vi "Transcriptor LabVIEW to C code 2.vi"(7 "vi path":path, 8 "Error In":errorcluster, 11 "Diagram in":refnum<vi>) -> (0 "Error Out":errorcluster, 1 "output cluster":T1, 2 "transcripted code":string, 3 "Diagram out":refnum<vi>)   [LabVIEW 2014]
panel:
  out "Cluster typedef[]":string[](array[string])
  out "FiringOrder":string[](array[string])
  out "Diagram wires declarations":string[](array[string])
  # "0. create definitions (ClusterConstant)\n1. get all wires and create their declarations\n2. if wires are connected to control or constant assign value to them\n3. translate elements of diagram by firing order\n4. assign values to outputs"
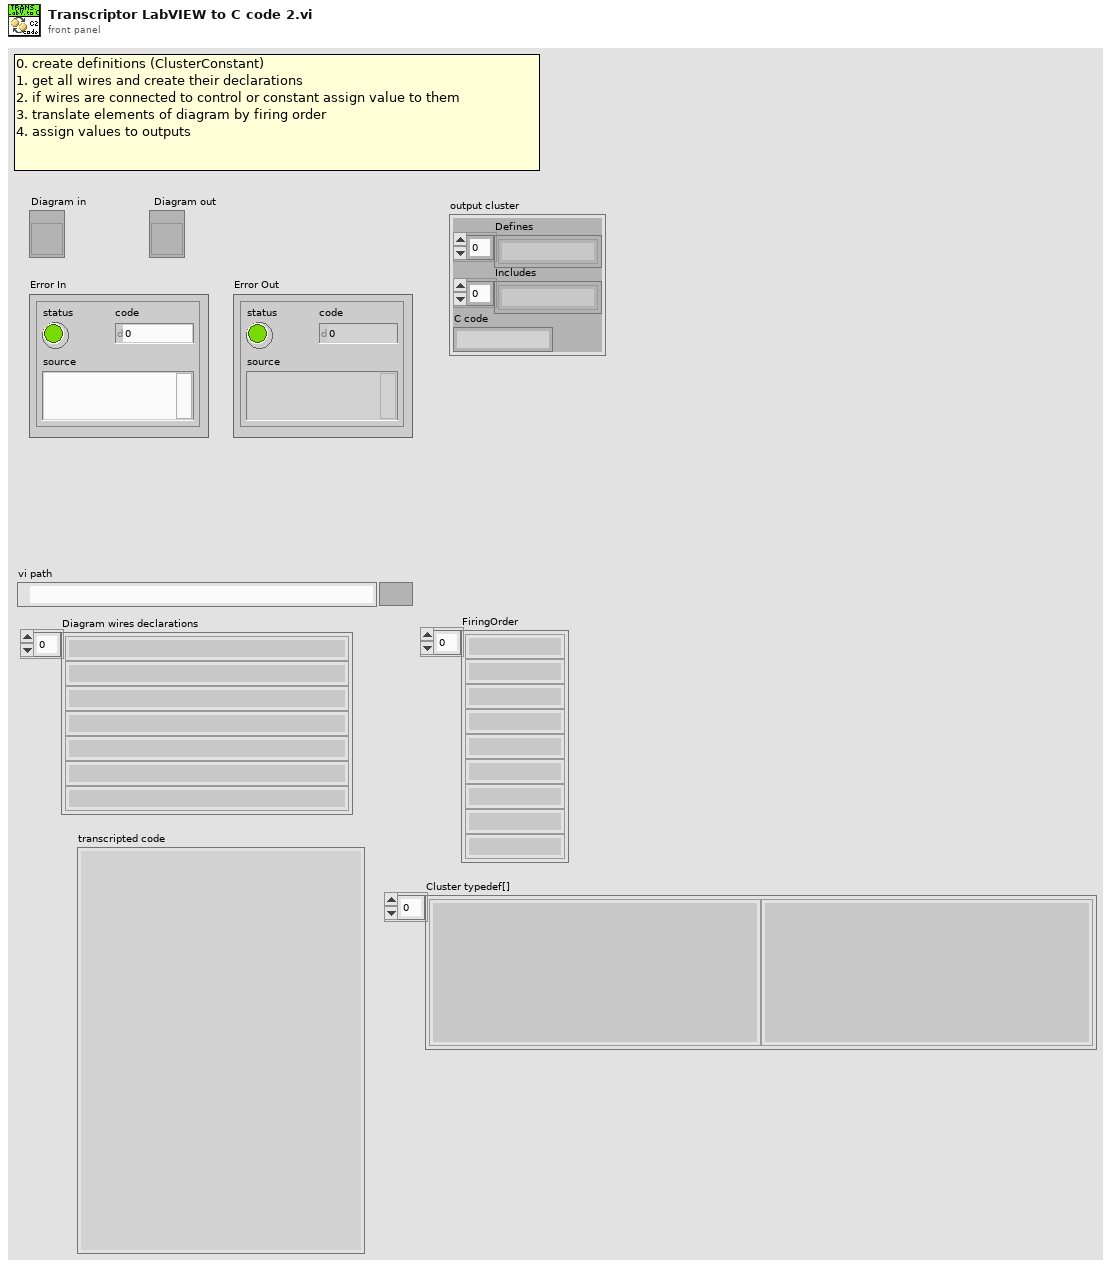
[diagram p1: front panel]
types:
  T1 = cluster{"Defines":string[], "Includes":string[], "C code":string}
  T2 = cluster{"wire labels":string[], "wire terminals datatypes":string[][]}
  T3 = cluster{"Defines":string[], "Includes":string[], "C code":string}[]
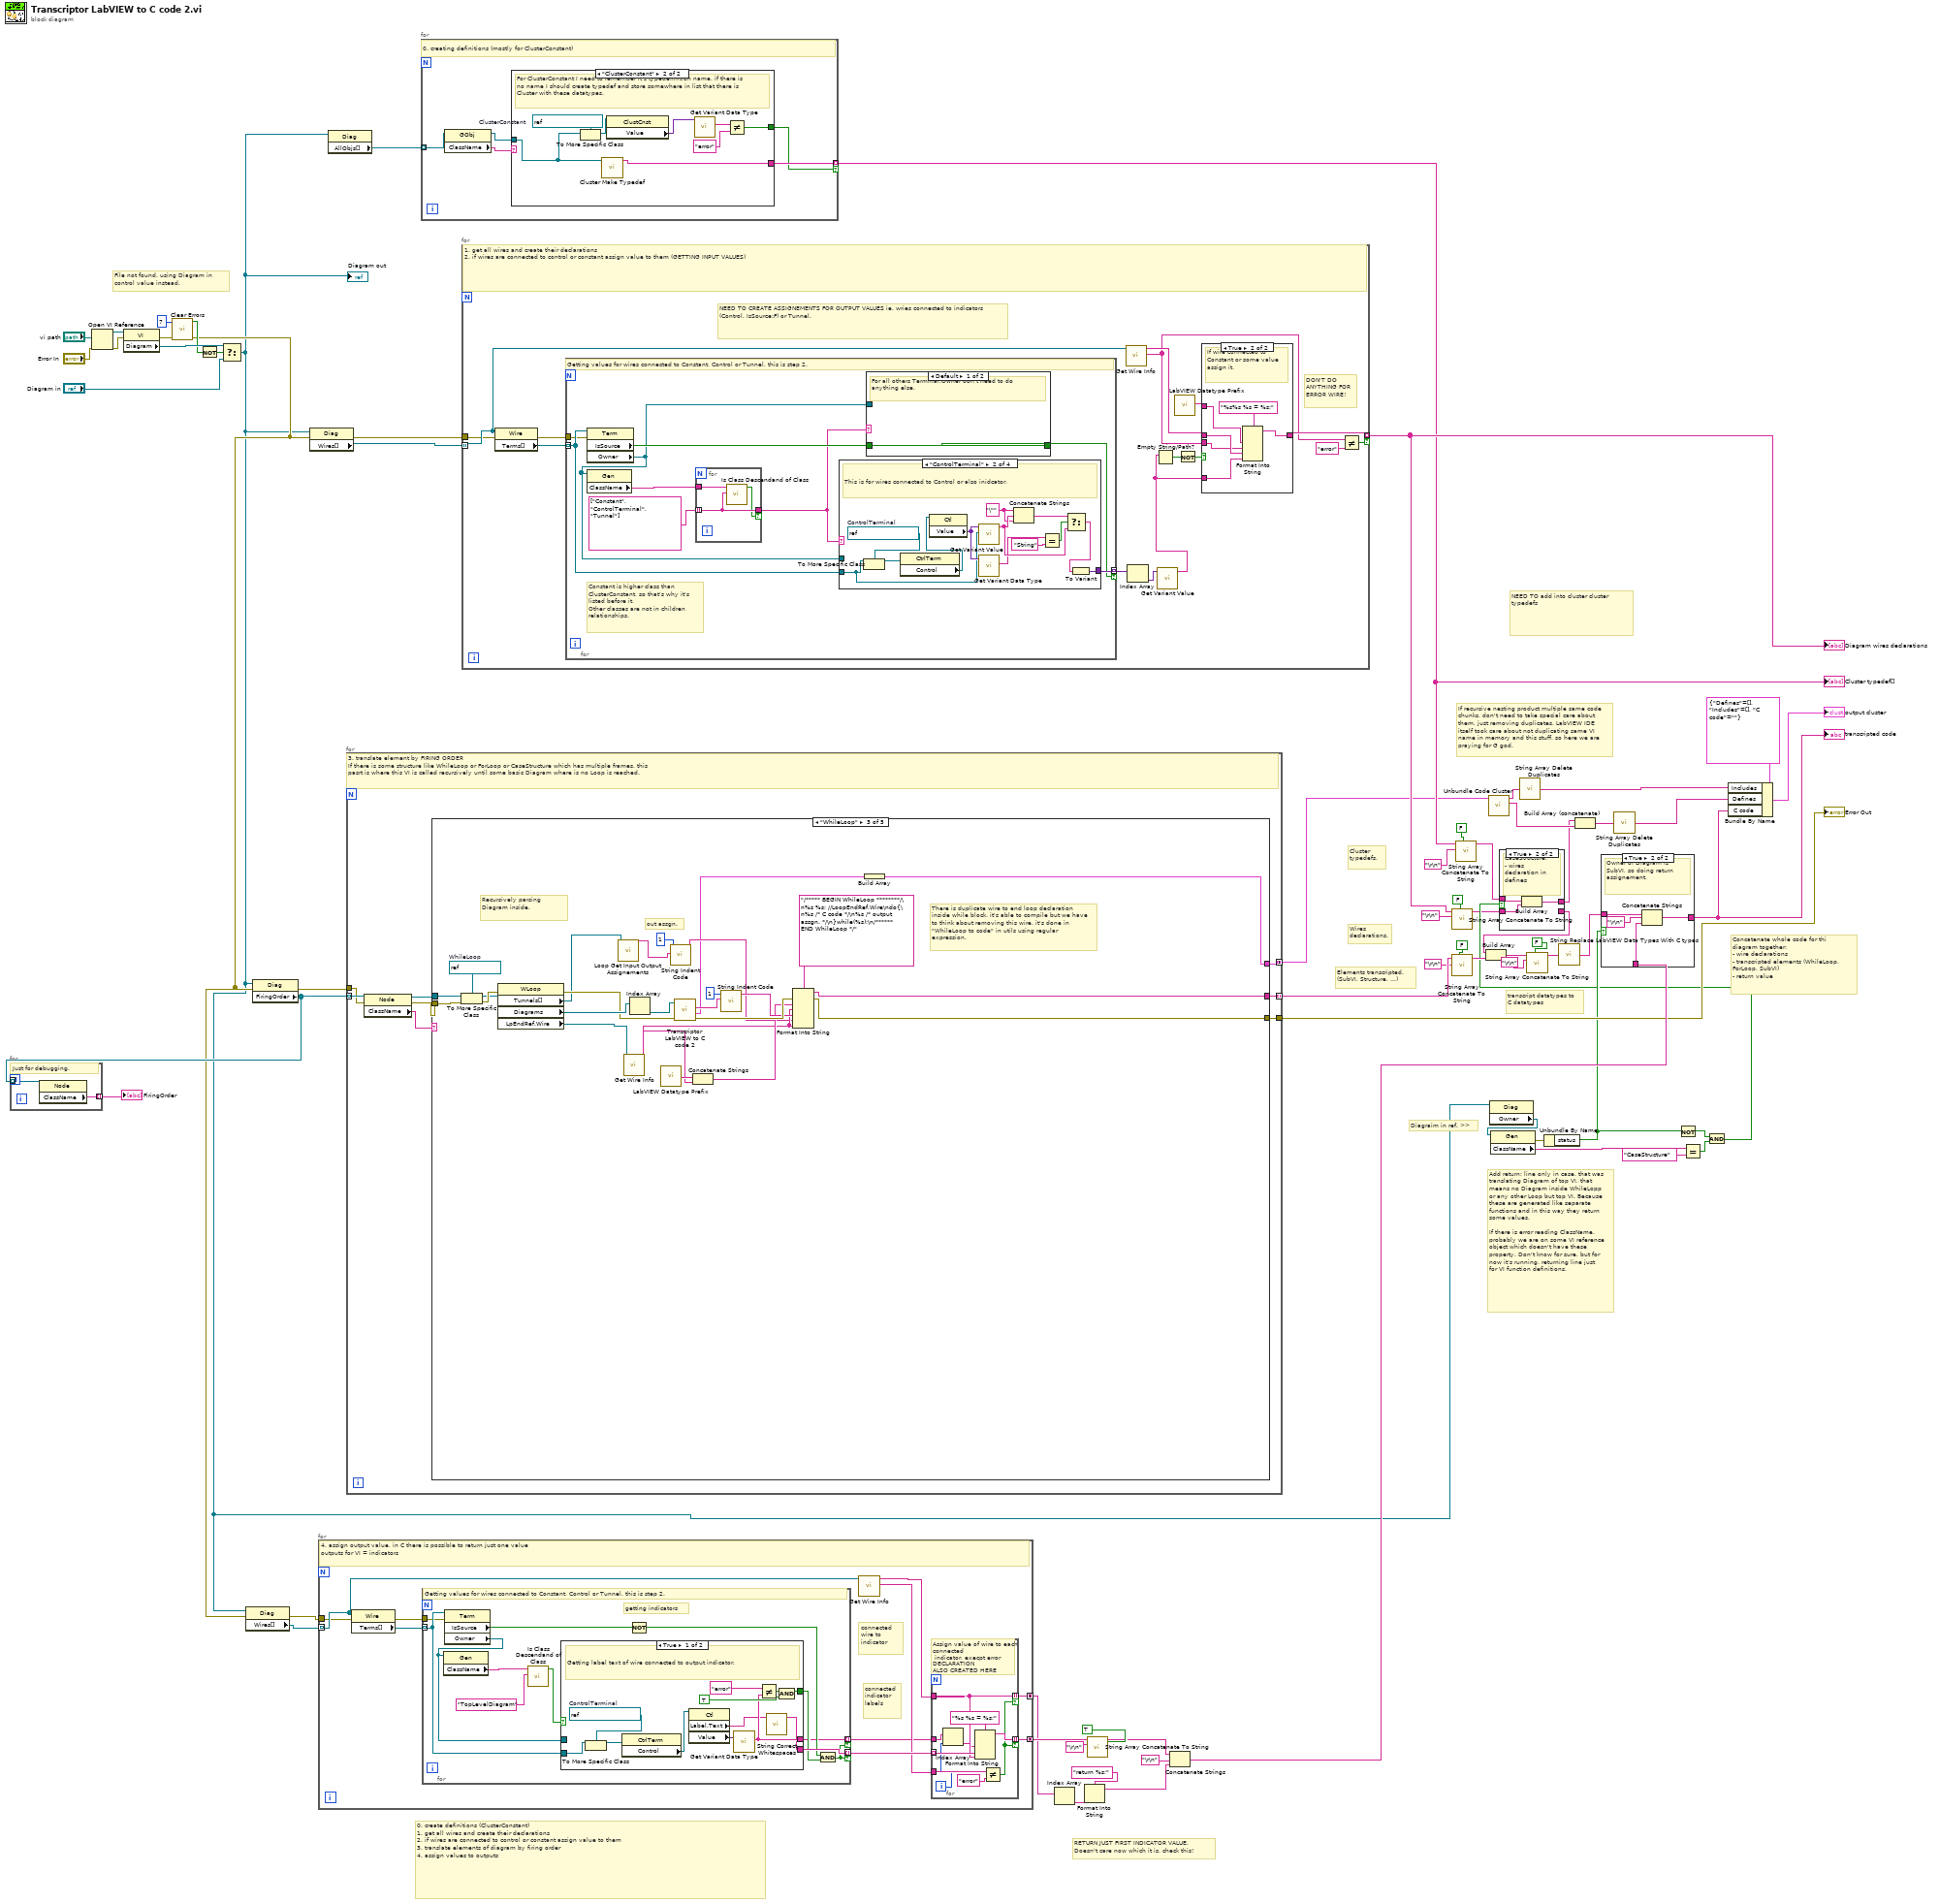
[diagram p0: block diagram]
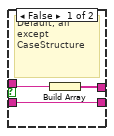
[diagram p2: hidden frame]
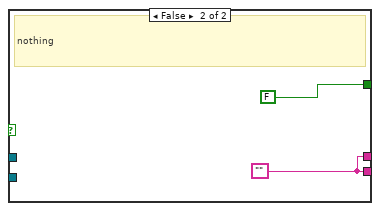
[diagram p4: hidden frame]
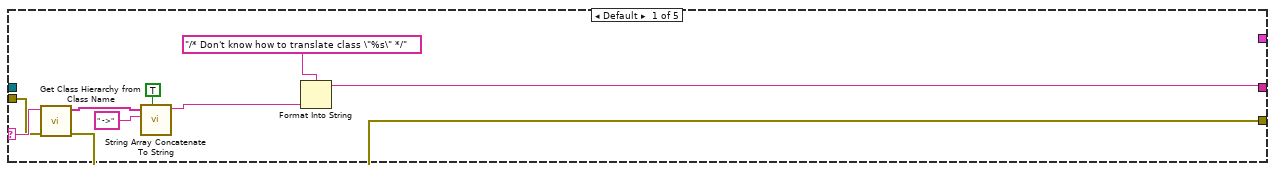
[diagram p6: hidden frame]
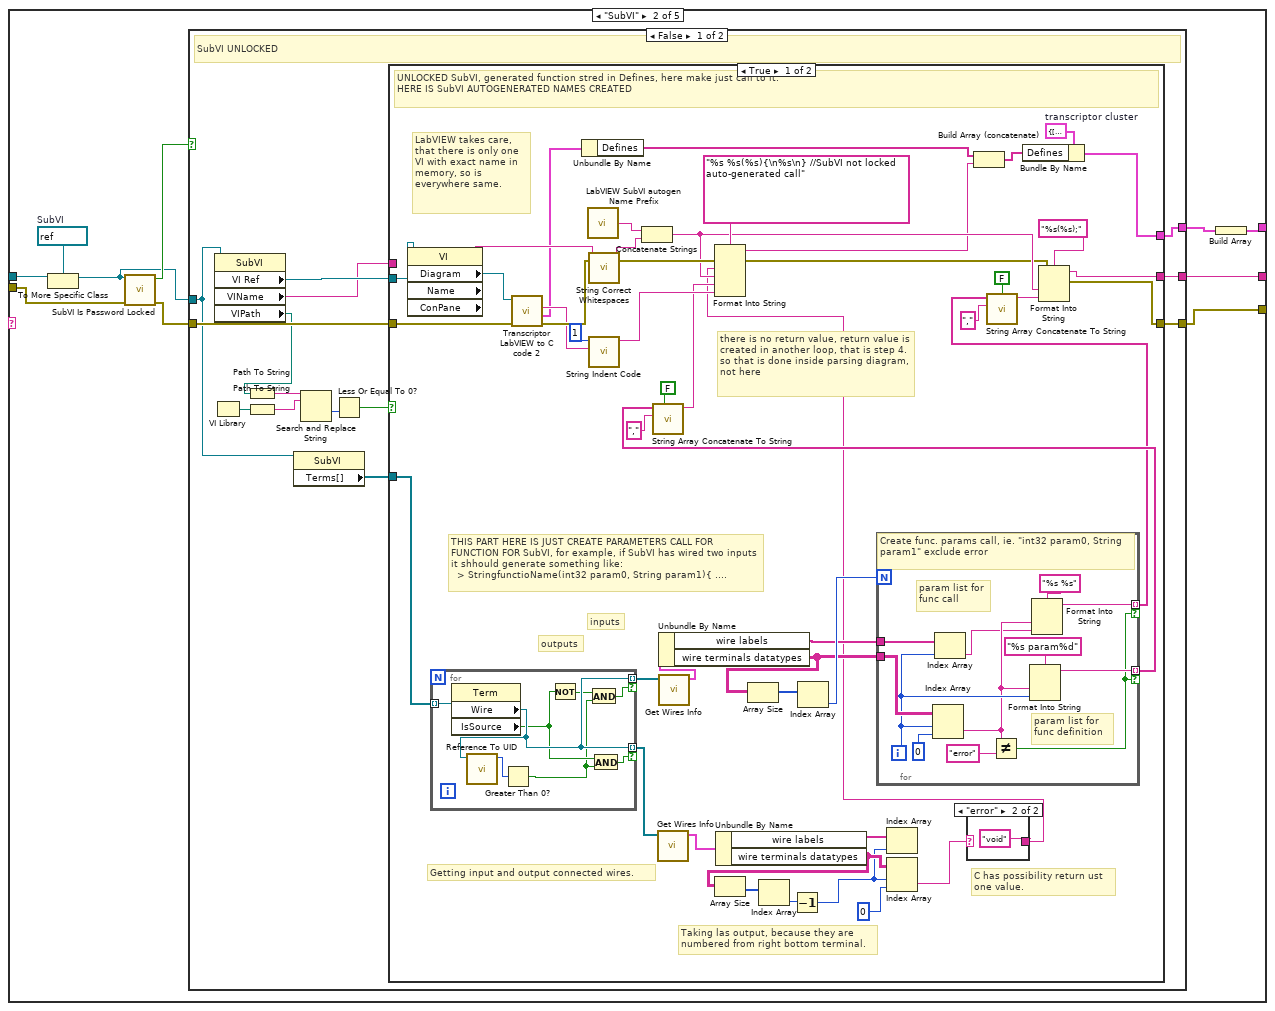
[diagram p7: hidden frame]
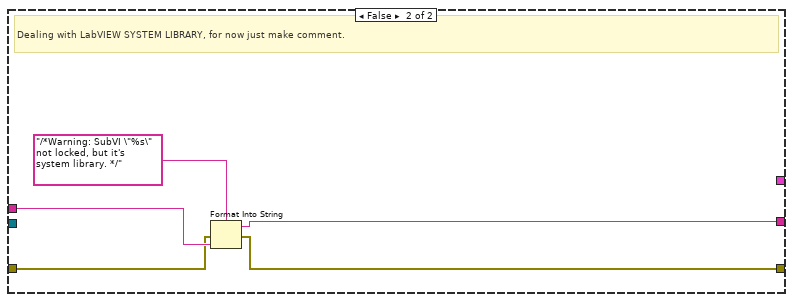
[diagram p9: hidden frame]
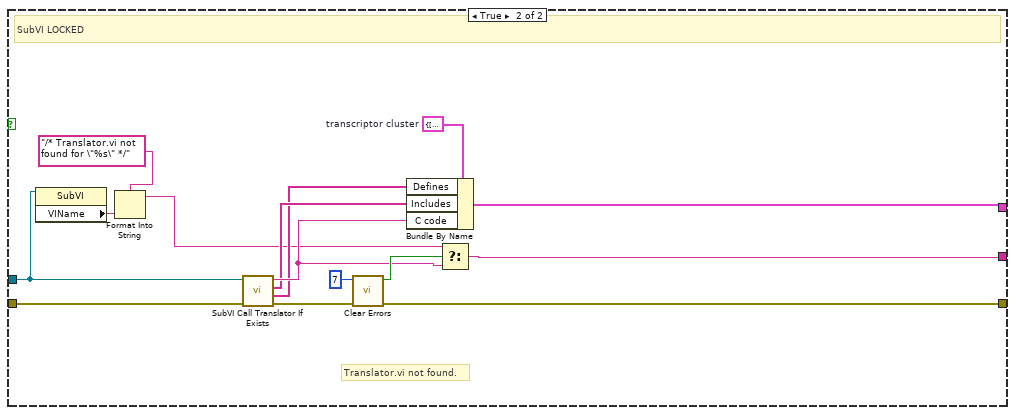
[diagram p10: hidden frame]
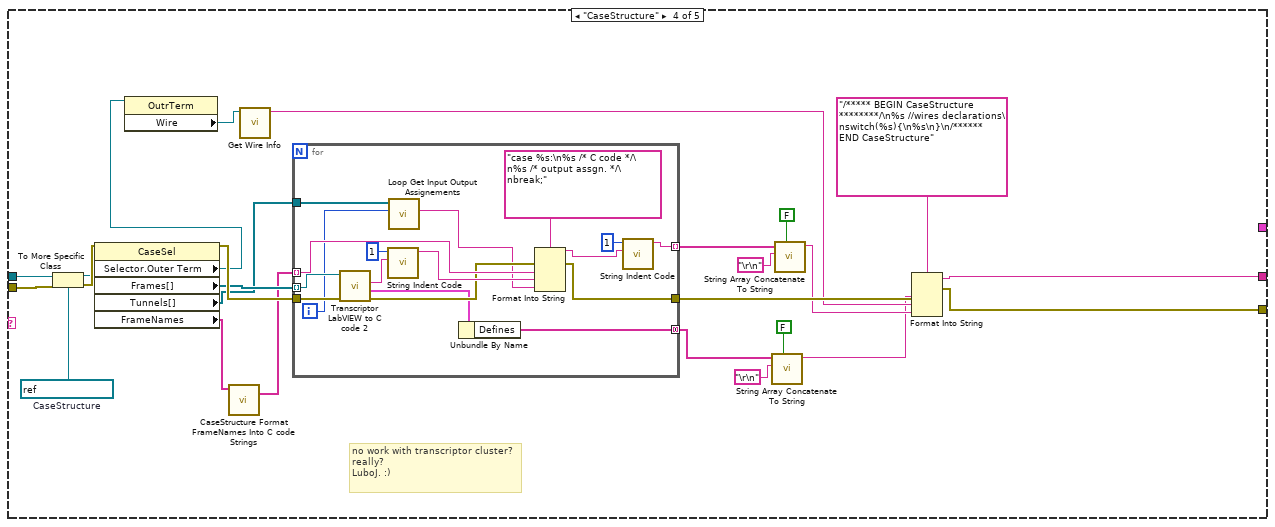
[diagram p11: hidden frame]
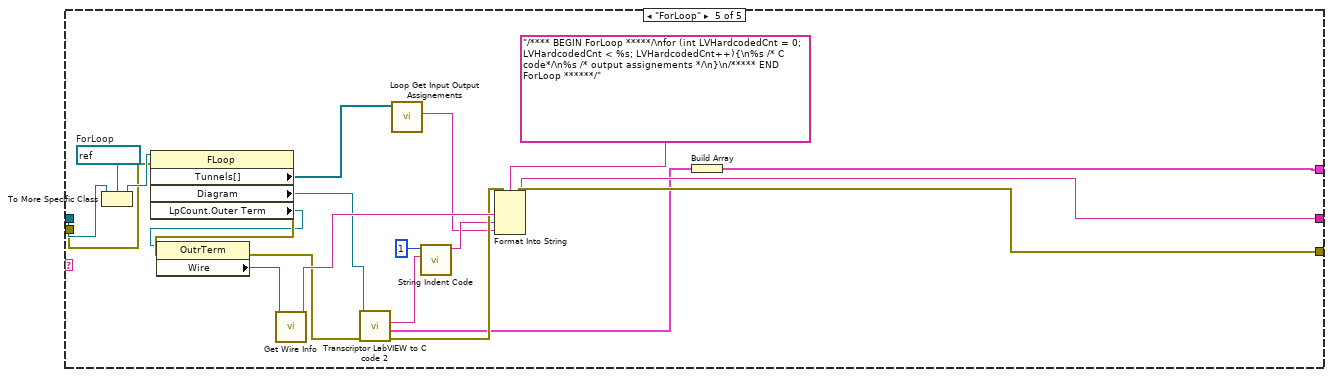
[diagram p12: hidden frame]
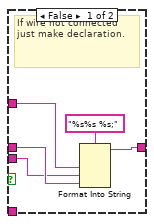
[diagram p13: hidden frame]
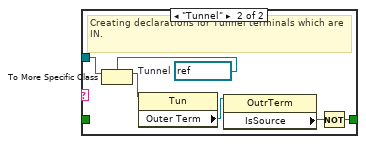
[diagram p14: hidden frame]
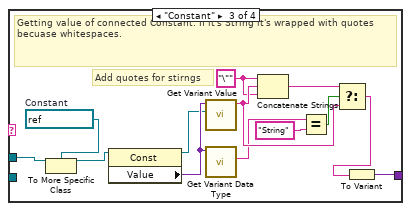
[diagram p16: hidden frame]
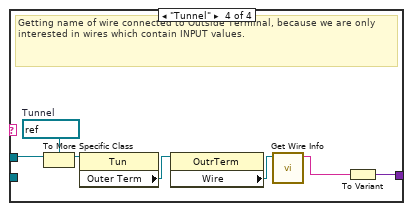
[diagram p17: hidden frame]
diagram:
  # "Diagraim in ref. >>"
  # "Add return; line only in case, that was translating Diagram of top VI, that means no Diagram inside WhileLopp or any other Loop but top VI. Because these are generated like separate functions and in this way they return some values.\n\nIf there is error reading ClassName, probably we are on some VI reference object which doesn't have these property. Don't know for sure, but for now it's running, returning line just for VI function definitions."
  # "RETURN JUST FIRST INDICATOR VALUE.\nDoesn't care now which it is, check this!"
  # "Concatenate whole code for thi diagram together:\n- wire declarations\n- transcripted elements (WhileLoop, ForLoop, SubVI)\n- return value"
  # "0. create definitions (ClusterConstant)\n1. get all wires and create their declarations\n2. if wires are connected to control or constant assign value to them\n3. translate elements of diagram by firing order\n4. assign values to outputs"
  # "If recursive nesting product multiple same code chunks, don't need to take special care about them, just removing duplicates, LabVIEW IDE itself took care about not duplicating same VI name in memory and this stuff, so here we are praying for G god."
  # "NEED TO add into cluster cluster typedefs"
  # "transcript datatypes to C datatypes"
  # "Elements transcripted.\n(SubVI, Structure, ...)"
  # "Wires declarations."
  # "Cluster typedefs."
  # "File not found, using Diagram in control value instead."
  n1 = Open VI Reference(vi path="vi path", error in (no error)="Error In") -> (vi reference=w66:refnum<vi>, error out=w65:errorcluster)  [unwired: 4 in]
  n2 = property class="VI"(reference=w66, error in=w65) -> (error out=w50:errorcluster, "Diagram"=w54:refnum<vi>)  [unwired: 1 out]
  n3 = call <vilib>:"Clear Errors.vi"("error in (no error)"=w50, "specific error code to clear (0: all)"=7) -> ("error out"=w29:errorcluster, "specific error cleared?"=w48:bool)  [unwired: 4 in]
  n4 = Not(x=w48) -> (.not. x?=w47:bool)
  n5 = Select(t=w54, s=w47, f="Diagram in") -> (s? t:f=w13:refnum<vi>)
  "Diagram out" <- w13
  n6 = property class="Diag"(reference=w13, error in=w29) -> (error out=w30:errorcluster, "Wires[]"=w31:refnum<vi>[])  [unwired: 1 out]
  n7 = property class="Diag"(reference=w13, error in=w29) -> (error out=w62:errorcluster, "FiringOrder"=w52:refnum<vi>[])  [unwired: 1 out]
  n8 = for {
    tunnel: w52 -> [w69] mode=indexing
    tunnel: [w68] -> w51 mode=indexing
    # "Just for debugging."
    n9 = property class="Node"(reference=w69) -> ("ClassName"=w68:string)  [unwired: 1 in, 2 out]
  }
  "FiringOrder" <- w51
  n10 = property class="Diag"(reference=w13, error in=w29) -> (error out=w63:errorcluster, "Wires[]"=w64:refnum<vi>[])  [unwired: 1 out]
  n11 = for {
    tunnel: w31 -> [w78] mode=indexing
    tunnel: w30 -> [w77]
    tunnel: [w73] -> w25 mode=concatenating
    tunnel: [w72] -> w23 mode=concatenating
    # "connected indicator labels"
    # "connected wire to indicator"
    # "4. assign output value, in C there is possible to return just one value\noutputs for VI = indicators"
    n12 = property class="Wire"(reference=w78, error in=w77) -> (error out=w76:errorcluster, "Terms[]"=w79:refnum<vi>[])  [unwired: 1 out]
    n13 = for {
      tunnel: w79 -> [w101] mode=indexing
      tunnel: [w94] -> w75 mode=indexing if=w90
      tunnel: w76 -> [w100]
      tunnel: [w91] -> w70 mode=indexing if=w90
      # "getting indicators"
      # "Getting values for wires connected to Constant, Control or Tunnel, this is step 2."
      n14 = property class="Term"(reference=w101, error in=w100) -> ("IsSource"=w99:bool, "Owner"=w98:refnum<vi>)  [unwired: 2 out]
      n15 = property class="Gen"(reference=w98) -> ("ClassName"=w97:string)  [unwired: 1 in, 2 out]
      n16 = call "Is Class Descendand of Class.vi"("Parent ClassName"="TopLevelDiagram", "ClassName"=w97) -> ("is Class descendant?"=w95:bool)  [unwired: 8 in, 1 out]
      n17 = case shown="True" w95 {
        tunnel: w98 -> [_ _]
        tunnel: w101 -> [w110 _]
        tunnel: [w102 w114] -> w94
        tunnel: [w105 FALSE] -> w92
        tunnel: [w104 w114] -> w91
        frame True {
          w113 = refnum<vi> refnum  # ControlTerminal
          # "Getting label text of wire connected to output indicator."
          n18 = To More Specific Class(target class=w113, reference=w110) -> (specific class reference=w112:refnum<vi>)  [unwired: 1 in, 1 out]
          n19 = property class="CtrlTerm"(reference=w112) -> ("Control"=w111:refnum<vi>)  [unwired: 1 in, 2 out]
          n20 = property class="Ctl"(reference=w111) -> ("Label.Text"=w103:string, "Value"=w109:variant)  [unwired: 1 in, 2 out]
          n21 = call "Get Variant Data Type.vi"("Variant in"=w109) -> ("first data type"=w104:string)  [unwired: 9 in, 1 out]
          n22 = Not Equal?(x="error", y=w104) -> (x != y?=w107:bool)
          n23 = call "String Correct Whitespaces.vi"("String in"=w103) -> ("String out"=w102:string)  [unwired: 10 in]
          n24 = And(x=w107, y=TRUE) -> (x .and. y?=w105:bool)
        }
        frame False {
          w114 = ""
          # "nothing"
        }
      }
      n25 = Not(x=w99) -> (.not. x?=w93:bool)
      n26 = And(x=w93, y=w92) -> (x .and. y?=w90:bool)
    }
    n27 = call "Get Wire Info.vi"("Wire"=w78) -> ("wire datatype"=w71:string, "wire label"=w74:string)  [unwired: 9 in]
    n28 = for {
      tunnel: w75 -> [w88] mode=indexing
      tunnel: w74 -> [w86]
      tunnel: [w87] -> w73 mode=indexing if=w83
      tunnel: [w86] -> w72 mode=indexing if=w83
      tunnel: w71 -> [w85]
      tunnel: w70 -> [w81]
      i -> [w82]
      # "Assign value of wire to each connected\n indicator, execpt error\nDECLARATION\nALSO CREATED HERE"
      n29 = Index Array(array=w81, index=w82) -> (element=w80:string)
      n30 = Format Into String(format string="%s %s = %s;", w80, w88, w86) -> (resulting string=w87:string)  [unwired: 2 in, 1 out]
      n31 = Not Equal?(x=w85, y="error" ("format string")) -> (x != y?=w83:bool)
    }
  }
  n32 = property class="Diag"(reference=w13) -> ("AllObjs[]"=w40:refnum<vi>[])  [unwired: 1 in, 2 out]
  n33 = for {
    tunnel: w52 -> [w123] mode=indexing
    tunnel: w62 -> [w121]
    tunnel: [w119] -> w61 mode=indexing
    tunnel: [w117] -> w14
    tunnel: [w116] -> w15 mode=concatenating
    # "3. translate element by FIRING ORDER\nIf there is some structure like WhileLoop or ForLoop or CaseStructure which has multiple frames, this\npasrt is where this VI is called recursively until some basic Diagram where is no Loop is reached."
    n34 = property class="Node"(reference=w123, error in=w121) -> (reference out=w120:refnum<vi>, error out=w118:errorcluster, "ClassName"=w122:string)
    n35 = case shown="\"WhileLoop\"" w122 {
      selector: w122 -> [w130 _ _ _ _]
      tunnel: w120 -> [_ w142 w271 w278 w334]
      tunnel: [w131 w138 w263 w291 w324] -> w119
      tunnel: w118 -> [w125 w137 w267 w294 w331]
      tunnel: [w124 w135 w261 w289 w325] -> w117
      tunnel: [_ w133 w254 _ w315] -> w116
      frame Default {
        n36 = call <vilib>:"Get Class Hierarchy from Class Name.vi"("error in (no error)"=w125, "Class Name"=w130) -> ("error out"=w124:errorcluster, "Class Hierarchy"=w128:string[])  [unwired: 8 in]
        n37 = call "String Array Concatenate To String.vi"("insert last delimiter?"=TRUE, "Delimiter char"=" ->", "Array String In"=w128) -> ("String"=w126:string)  [unwired: 8 in]
        n38 = Format Into String(format string="/* Don't know how to translate class \"%s\" */", w126) -> (resulting string=w131:string)  [unwired: 2 in, 1 out]
      }
      frame "SubVI" {
        w141 = refnum<vi> refnum  # SubVI
        n39 = To More Specific Class(target class=w141, reference=w142) -> (specific class reference=w139:refnum<vi>)  [unwired: 1 in, 1 out]
        n40 = call "SubVI Is Password Locked.vi"("Error In"=w137, "SubVI ref"=w139) -> ("Error Out"=w136:errorcluster, "isPasswordLocked?"=w140:bool)  [unwired: 8 in]
        n41 = case shown="False" w140 {
          tunnel: w139 -> [w145 w235]
          tunnel: [w154 w242] -> w138
          tunnel: w136 -> [w156 w241]
          tunnel: [w153 w240] -> w135
          tunnel: [w143 w231] -> w134
          frame False {
            # "SubVI UNLOCKED"
            n42 = VI Library() -> (path=w150:path)
            n43 = property class="SubVI"(reference=w145) -> ("VI Ref"=w155:refnum<vi>, "VIName"=w152:string, "VIPath"=w151:path)  [unwired: 1 in, 2 out]
            n44 = Path To String(path=w151) -> (string=w149:string)
            n45 = Path To String(path=w150) -> (string=w148:string)
            n46 = property class="SubVI"(reference=w145) -> ("Terms[]"=w144:refnum<vi>[])  [unwired: 1 in, 2 out]
            n47 = Search and Replace String(input string=w149, search string=w148) -> (number of replacements=w147:i32)  [unwired: 6 in, 3 out]
            n48 = Less Or Equal To 0?(x=w147) -> (x <= 0?=w146:bool)
            n49 = case shown="True" w146 {
              tunnel: w156 -> [w203 w226]
              tunnel: w155 -> [w186 _]
              tunnel: [w201 w229] -> w154
              tunnel: [w188 w228] -> w153
              tunnel: w152 -> [_ w227]
              tunnel: [w202 _] -> w143
              tunnel: w144 -> [w179 _]
              frame True {
                w159 = T1 {"Defines"=[], "Includes"=[], "C code"=""}  # transcriptor cluster
                # "THIS PART HERE IS JUST CREATE PARAMETERS CALL FOR FUNCTION FOR SubVI, for example, if SubVI has wired two inputs it shhould generate something like:\n  > StringfunctioName(int32 param0, String param1){ ...."
                # "there is no return value, return value is created in another loop, that is step 4.\nso that is done inside parsing diagram, not here"
                # "Taking las output, because they are numbered from right bottom terminal."
                # "outputs"
                # "inputs"
                # "Getting input and output connected wires."
                # "C has possibility return ust one value."
                # "LabVIEW takes care, that there is only one VI with exact name in memory, so is everywhere same."
                # "UNLOCKED SubVI, generated function stred in Defines, here make just call to it.\nHERE IS SubVI AUTOGENERATED NAMES CREATED"
                n50 = property class="VI" props=["Diagram", "Name", "ConPane"](reference=w186) -> ("Diagram"=w187:refnum<vi>, "Name"=w198:string)  [unwired: 1 in, 3 out]
                n51 = for {
                  tunnel: [w223] -> w177 mode=indexing if=w220
                  tunnel: [w223] -> w178 mode=indexing if=w221
                  tunnel: w179 -> [w225] mode=indexing
                  n52 = property class="Term"(reference=w225) -> ("Wire"=w223:refnum<vi>, "IsSource"=w219:bool)  [unwired: 1 in, 2 out]
                  n53 = call "Reference To UID.vi"("Reference"=w223) -> ("UID"=w224:i32)  [unwired: 10 in]
                  n54 = Greater Than 0?(x=w224) -> (x > 0?=w218:bool)
                  n55 = Not(x=w219) -> (.not. x?=w222:bool)
                  n56 = And(x=w222, y=w218) -> (x .and. y?=w221:bool)
                  n57 = And(x=w219, y=w218) -> (x .and. y?=w220:bool)
                }
                n58 = call "Transcriptor LabVIEW to C code 2.vi"("Error In"=w203, "Diagram in"=w187) -> ("Error Out"=w199:errorcluster, "output cluster"=w158:T1, "transcripted code"=w197:string)  [unwired: 6 in, 1 out]
                n59 = Unbundle By Name(w158) -> ("Defines"=w157:string[])
                n60 = call "LabVIEW SubVI autogen Name Prefix.vi"() -> ("datatype prefix"=w194:string)
                n61 = call "String Correct Whitespaces.vi"("String in"=w198) -> ("String out"=w193:string)  [unwired: 10 in]
                n62 = call "String Indent Code.vi"("complete code"=w197, "actual nested level"=1) -> ("indented code"=w183:string)  [unwired: 9 in]
                n63 = Concatenate Strings(w194, w193) -> (w192:string)
                n64 = call "Get Wires Info.vi"("connected\nwires refs."=w177) -> ("output cluster 2"=w181:T2)  [unwired: 10 in]
                n65 = call "Get Wires Info.vi"("connected\nwires refs."=w178) -> ("output cluster 2"=w176:T2)  [unwired: 10 in]
                n66 = Unbundle By Name(w176) -> ("wire labels"=w171:string[], "wire terminals datatypes"=w173:string[][])
                n67 = Unbundle By Name(w181) -> ("wire labels"=w180:string[], "wire terminals datatypes"=w163:string[][])
                n68 = Array Size(array=w163) -> (size(s)=w162:i32[])
                n69 = Array Size(array=w173) -> (size(s)=w175:i32[])
                n70 = Index Array(array=w162) -> (element=w161:i32)  [unwired: 1 in]
                n71 = Decrement(x=w161) -> (x-1=w160:i32)
                n72 = Index Array(array=w175) -> (element=w174:i32)  [unwired: 1 in]
                n73 = for {
                  N: w174 -> [_]
                  tunnel: w173 -> [w217]
                  tunnel: [w214] -> w172 mode=indexing if=w207
                  tunnel: w171 -> [w212]
                  tunnel: [w206] -> w167 mode=indexing if=w207
                  i -> [w211]
                  # "param list for\nfunc call"
                  # "param list for\nfunc definition"
                  # "Create func. params call, ie. \"int32 param0, String param1\" exclude error"
                  n74 = Index Array(array=w217, index (row)=w211, index (col)=0 ("disabled index (col)")) -> (element=w209:string)
                  n75 = Index Array(array=w212, index=w211) -> (element=w208:string)
                  n76 = Not Equal?(x=w209, y="error") -> (x != y?=w207:bool)
                  n77 = Format Into String(format string="%s param%d", w209, w211) -> (resulting string=w214:string)  [unwired: 2 in, 1 out]
                  n78 = Format Into String(format string="%s %s", w209, w208) -> (resulting string=w206:string)  [unwired: 2 in, 1 out]
                }
                n79 = call "String Array Concatenate To String.vi"("insert last delimiter?"=FALSE, "Delimiter char"=",", "Array String In"=w172) -> ("String"=w182:string)  [unwired: 8 in]
                n80 = Index Array(array=w180, index=w160) -> ()  [unwired: 1 out]
                n81 = Index Array(array=w163, index (row)=w160, index (col)=0 ("index (row)")) -> (element=w165:string)
                n82 = case shown="\"error\"" w165 {
                  selector: w165 -> [w204 _]
                  tunnel: [w204 "void" ("y")] -> w164
                  frame Default {
                  }
                  frame "error" {
                  }
                }
                n83 = Format Into String(format string="%s %s(%s){\n%s\n} //SubVI not locked auto-generated call", error in=w199, w164, w192, w182, w183) -> (resulting string=w190:string, error out=w189:errorcluster)  [unwired: 1 in]
                n84 = Build Array (concatenate)(w157, w190) -> (w191:string[])
                n85 = call "String Array Concatenate To String.vi"("insert last delimiter?"=FALSE, "Delimiter char"=",", "Array String In"=w167) -> ("String"=w169:string)  [unwired: 8 in]
                n86 = Bundle By Name(cluster=w159, "Defines"=w191) -> (w202:T1)
                n87 = Format Into String(format string="%s(%s);", error in=w189, w192, w169) -> (resulting string=w201:string, error out=w188:errorcluster)  [unwired: 1 in]
              }
              frame False {
                # "Dealing with LabVIEW SYSTEM LIBRARY, for now just make comment."
                n88 = Format Into String(format string="/*Warning: SubVI \"%s\" not locked, but it's system library. */", error in=w226, w227) -> (resulting string=w229:string, error out=w228:errorcluster)  [unwired: 1 in]
              }
            }
          }
          frame True {
            w239 = T1 {"Defines"=[], "Includes"=[], "C code"=""}  # transcriptor cluster
            # "Translator.vi not found."
            # "SubVI LOCKED"
            n89 = property class="SubVI"(reference=w235) -> ("VIName"=w234:string)  [unwired: 1 in, 2 out]
            n90 = Format Into String(format string="/* Translator.vi not found for \"%s\" */" ("t"), w234) -> (resulting string=w232:string)  [unwired: 2 in, 1 out]
            n91 = call "SubVI Call Translator If Exists.vi"("Error In"=w241, "SubVI Refnum"=w235) -> ("Error Out"=w245:errorcluster, "Defines"=w236:string[], "Includes"=w237:string[], "Replaced Code"=w238:string)  [unwired: 6 in]
            n92 = call <vilib>:"Clear Errors.vi"("error in (no error)"=w245, "specific error code to clear (0: all)"=7) -> ("error out"=w240:errorcluster, "specific error cleared?"=w243:bool)  [unwired: 4 in]
            n93 = Bundle By Name(cluster=w239, "Defines"=w236, "Includes"=w237, "C code"=w238) -> (w231:T1)
            n94 = Select(t=w232, s=w243, f=w238) -> (s? t:f=w242:string)
          }
        }
        n95 = Build Array(w134) -> (w133:T3)
      }
      frame "WhileLoop" {
        w270 = refnum<vi> refnum  # WhileLoop
        # "out assgn."
        # "There is duplicate wire to end loop declaration inside while block, it's able to compile but we have to think about removing this wire, it's done in \"WhileLoop to code\" in utils using regular expression."
        # "Recursively parsing Diagram inside."
        n96 = To More Specific Class(target class=w270, reference=w271, error in=w267) -> (specific class reference=w260:refnum<vi>, error out=w269:errorcluster)
        n97 = property class="WLoop"(reference=w260, error in=w269) -> (error out=w266:errorcluster, "Tunnels[]"=w255:refnum<vi>[], "Diagrams"=w268:refnum<vi>[], "LpEndRef.Wire"=w259:refnum<vi>)  [unwired: 1 out]
        n98 = call "Loop Get Input Output Assignements.vi"("Loop Tunnels[]"=w255) -> ("Output assignements"=w248:string)  [unwired: 9 in, 1 out]
        n99 = call "Get Wire Info.vi"("Wire"=w259) -> ("wire datatype"=w252:string, "wire label"=w250:string)  [unwired: 9 in]
        n100 = Index Array(array=w268) -> (element=w265:refnum<vi>)  [unwired: 1 in]
        n101 = call "LabVIEW Datatype Prefix.vi"() -> ("datatype prefix"=w253:string)
        n102 = call "String Indent Code.vi"("complete code"=w248, "actual nested level"=1) -> ("indented code"=w247:string)  [unwired: 9 in]
        n103 = call "Transcriptor LabVIEW to C code 2.vi"("Error In"=w266, "Diagram in"=w265) -> ("Error Out"=w262:errorcluster, "output cluster"=w246:T1, "transcripted code"=w258:string)  [unwired: 6 in, 1 out]
        n104 = Concatenate Strings(w253, w252) -> (w251:string)
        n105 = call "String Indent Code.vi"("complete code"=w258, "actual nested level"=1) -> ("indented code"=w256:string)  [unwired: 9 in]
        n106 = Format Into String(format string="/***** BEGIN WhileLoop ********/\n%s %s; //LoopEndRef.Wire\ndo{\n%s /* C code */\n%s /* output assgn. */\n}while(%s);\n/****** END WhileLoop */", error in=w262, w251, w250, w256, w247, w250) -> (resulting string=w263:string, error out=w261:errorcluster)  [unwired: 1 in]
        n107 = Build Array(w246) -> (w254:T3)
      }
      frame "CaseStructure" {
        w296 = refnum<vi> refnum  # CaseStructure
        # "no work with transcriptor cluster? really?\nLuboJ. :)"
        n108 = To More Specific Class(target class=w296, reference=w278, error in=w294) -> (specific class reference=w288:refnum<vi>, error out=w295:errorcluster)
        n109 = property class="CaseSel"(reference=w288, error in=w295) -> (error out=w293:errorcluster, "Selector.Outer Term"=w286:refnum<vi>, "Frames[]"=w287:refnum<vi>[], "Tunnels[]"=w279:refnum<vi>[], "FrameNames"=w276:string[])  [unwired: 1 out]
        n110 = property class="OutrTerm"(reference=w286) -> ("Wire"=w285:refnum<vi>)  [unwired: 1 in, 2 out]
        n111 = call "CaseStructure Format FrameNames Into C code Strings.vi"("FrameNames in"=w276) -> ("c code cases names"=w277:string[])  [unwired: 10 in]
        n112 = call "Get Wire Info.vi"("Wire"=w285) -> ("wire label"=w284:string)  [unwired: 9 in, 1 out]
        n113 = for {
          tunnel: w293 -> [w313]
          tunnel: [w305] -> w290
          tunnel: w287 -> [w312] mode=indexing
          tunnel: w277 -> [w308] mode=indexing
          tunnel: [w303] -> w281 mode=indexing
          tunnel: w279 -> [w300]
          tunnel: [w297] -> w273 mode=concatenating
          i -> [w301]
          n114 = call "Transcriptor LabVIEW to C code 2.vi"("Error In"=w313, "Diagram in"=w312) -> ("Error Out"=w306:errorcluster, "output cluster"=w298:T1, "transcripted code"=w310:string)  [unwired: 6 in, 1 out]
          n115 = call "String Indent Code.vi"("complete code"=w310, "actual nested level"=1) -> ("indented code"=w309:string)  [unwired: 9 in]
          n116 = call "Loop Get Input Output Assignements.vi"("Inside Terms[] offset"=w301, "Loop Tunnels[]"=w300) -> ("Output assignements"=w299:string)  [unwired: 8 in, 1 out]
          n117 = Unbundle By Name(w298) -> ("Defines"=w297:string[])
          n118 = Format Into String(format string="case %s:\n%s /* C code */\n%s /* output assgn. */\nbreak;", error in=w306, w308, w309, w299) -> (resulting string=w302:string, error out=w305:errorcluster)  [unwired: 1 in]
          n119 = call "String Indent Code.vi"("complete code"=w302, "actual nested level"=1) -> ("indented code"=w303:string)  [unwired: 9 in]
        }
        n120 = call "String Array Concatenate To String.vi"("insert last delimiter?"=FALSE, "Delimiter char"="\r\n", "Array String In"=w273) -> ("String"=w272:string)  [unwired: 8 in]
        n121 = call "String Array Concatenate To String.vi"("insert last delimiter?"=FALSE, "Delimiter char"="\r\n", "Array String In"=w281) -> ("String"=w280:string)  [unwired: 8 in]
        n122 = Format Into String(format string="/***** BEGIN CaseStructure ********/\n%s //wires declarations\nswitch(%s){\n%s\n}\n/****** END CaseStructure", error in=w290, w272, w284, w280) -> (resulting string=w291:string, error out=w289:errorcluster)  [unwired: 1 in]
      }
      frame "ForLoop" {
        w333 = refnum<vi> refnum  # ForLoop
        n123 = To More Specific Class(target class=w333, reference=w334) -> (specific class reference=w332:refnum<vi>)  [unwired: 1 in, 1 out]
        n124 = property class="FLoop"(reference=w332, error in=w331) -> (error out=w330:errorcluster, "Tunnels[]"=w317:refnum<vi>[], "Diagram"=w323:refnum<vi>, "LpCount.Outer Term"=w329:refnum<vi>)  [unwired: 1 out]
        n125 = property class="OutrTerm"(reference=w329, error in=w330) -> (error out=w322:errorcluster, "Wire"=w328:refnum<vi>)  [unwired: 1 out]
        n126 = call "Get Wire Info.vi"("Wire"=w328) -> ("wire label"=w326:string)  [unwired: 9 in, 1 out]
        n127 = call "Transcriptor LabVIEW to C code 2.vi"("Error In"=w322, "Diagram in"=w323) -> ("Error Out"=w321:errorcluster, "output cluster"=w314:T1, "transcripted code"=w320:string)  [unwired: 6 in, 1 out]
        n128 = call "Loop Get Input Output Assignements.vi"("Loop Tunnels[]"=w317) -> ("Output assignements"=w316:string)  [unwired: 9 in, 1 out]
        n129 = call "String Indent Code.vi"("complete code"=w320, "actual nested level"=1) -> ("indented code"=w318:string)  [unwired: 9 in]
        n130 = Format Into String(format string="/**** BEGIN ForLoop *****/\nfor (int LVHardcodedCnt = 0;  LVHardcodedCnt < %s; LVHardcodedCnt++){\n%s /* C code*/\n%s /* output assignements */\n}\n/***** END ForLoop ******/", error in=w321, w326, w318, w316) -> (resulting string=w324:string, error out=w325:errorcluster)  [unwired: 1 in]
        n131 = Build Array(w314) -> (w315:T3)
      }
    }
  }
  "Error Out" <- w14
  n132 = for {
    tunnel: w40 -> [w339] mode=indexing
    tunnel: [w336] -> w37 mode=indexing if=w335
    # "0. creating definitions (mostly for ClusterConstant)"
    n133 = property class="GObj"(reference=w339) -> (reference out=w337:refnum<vi>, "ClassName"=w338:string)  [unwired: 1 in, 1 out]
    n134 = case shown="\"ClusterConstant\"" w338 {
      tunnel: w337 -> [_ w342]
      tunnel: [_ w340] -> w336
      tunnel: [_ w344] -> w335
      frame Default {
        # "If wire is not wired to anything from what I have to read value, output is default Variant value (hope that is empty Variant), and there will be just wire declaration without assignement in generated code."
      }
      frame "ClusterConstant" {
        w343 = refnum<vi> refnum  # ClusterConstant
        # "For ClusterConstant I need to remember it's typedefinition name, if there is no name I should create typedef and store somewhere in list that there is Cluster with these datatypes."
        n135 = To More Specific Class(target class=w343, reference=w342) -> (specific class reference=w341:refnum<vi>)  [unwired: 1 in, 1 out]
        n136 = call "Cluster Make Typedef.vi"("GObject in"=w342) -> ("String"=w340:string)  [unwired: 10 in]
        n137 = property on="Property Node" class="ClustCnst"(reference=w341) -> ("Value"=w347:variant)  [unwired: 1 in, 2 out]
        n138 = call "Get Variant Data Type.vi"("Variant in"=w347) -> ("first data type"=w346:string)  [unwired: 9 in, 1 out]
        n139 = Not Equal?(x=w346, y="error") -> (x != y?=w344:bool)
      }
    }
  }
  "Cluster typedef[]" <- w37
  n140 = for {
    tunnel: w64 -> [w360] mode=indexing
    tunnel: [w357] -> w56 mode=indexing if=w353
    tunnel: w63 -> [w350]
    # "NEED TO CREATE ASSIGNEMENTS FOR OUTPUT VALUES ie. wries connected to indicators (Control, IsSource:F) or Tunnel."
    # "DON'T DO ANYTHING FOR ERROR WIRE!"
    # "1. get all wires and create their declarations\n2. if wires are connected to control or constant assign value to them (GETTING INPUT VALUES)"
    n141 = property class="Wire"(reference=w360, error in=w350) -> (error out=w349:errorcluster, "Terms[]"=w362:refnum<vi>[])  [unwired: 1 out]
    n142 = for {
      tunnel: w362 -> [w381] mode=indexing
      tunnel: [w382] -> w361 mode=indexing if=w379
      tunnel: w349 -> [w380]
      # "Constant is higher class than ClusterConstant, so that's why it's listed before it.\nOther classes are not in children relationships."
      # "Getting values for wires connected to Constant, Control or Tunnel, this is step 2."
      n143 = property class="Term"(reference=w381, error in=w380) -> ("IsSource"=w378:bool, "Owner"=w377:refnum<vi>)  [unwired: 2 out]
      n144 = property class="Gen"(reference=w377) -> ("ClassName"=w375:string)  [unwired: 1 in, 2 out]
      n145 = for {
        tunnel: string[] ["Constant", "ControlTerminal", "Tunnel"] -> [w384] mode=indexing
        tunnel: w375 -> [w385]
        tunnel: [w384] -> w374 if=w383
        n146 = call "Is Class Descendand of Class.vi"("Parent ClassName"=w384, "ClassName"=w385) -> ("is Class descendant?"=w383:bool)  [unwired: 8 in, 1 out]
      }
      n147 = case shown="\"ControlTerminal\"" w374 {
        tunnel: w377 -> [_ _ w418 w423]
        tunnel: [_ w394 w408 w424] -> w382
        tunnel: w381 -> [_ w393 _ _]
        frame Default {
          # "If wire is not wired to anything from what I have to read value, output is default Variant value (hope that is empty Variant), and there will be just wire declaration without assignement in generated code."
        }
        frame "ControlTerminal" {
          w399 = "\"" ("string")
          w405 = refnum<vi> refnum  # ControlTerminal
          # "This is for wires connected to Control or also inidcator."
          n148 = To More Specific Class(target class=w405, reference=w393) -> (specific class reference=w404:refnum<vi>)  [unwired: 1 in, 1 out]
          n149 = property class="CtrlTerm"(reference=w404) -> ("Control"=w403:refnum<vi>)  [unwired: 1 in, 2 out]
          n150 = property class="Ctl"(reference=w403) -> ("Value"=w395:variant)  [unwired: 1 in, 2 out]
          n151 = call "Get Variant Value.vi"("GObj Refnum"=w393, "Variant in"=w395) -> ("Variant value as string"=w401:string)  [unwired: 9 in]
          n152 = call "Get Variant Data Type.vi"("Variant in"=w395) -> ("first data type"=w397:string)  [unwired: 9 in, 1 out]
          n153 = Concatenate Strings(w399, w401, w399) -> (w402:string)
          n154 = Equal?(x=w397, y="String") -> (x = y?=w400:bool)
          n155 = Select(t=w402, s=w400, f=w401) -> (s? t:f=w396:string)
          n156 = To Variant(anything=w396) -> (Variant=w394:variant)
        }
        frame "Constant" {
          w412 = "\"" ("string")
          w417 = refnum<vi> refnum  # Constant
          # "Add quotes for stirngs"
          # "Getting value of connected Constant. If it's String it's wrapped with quotes becuase whitespaces."
          n157 = To More Specific Class(target class=w417, reference=w418) -> (specific class reference=w416:refnum<vi>)  [unwired: 1 in, 1 out]
          n158 = property class="Const"(reference=w416) -> (reference out=w406:refnum<vi>, "Value"=w409:variant)  [unwired: 1 in, 1 out]
          n159 = call "Get Variant Value.vi"("GObj Refnum"=w406, "Variant in"=w409) -> ("Variant value as string"=w414:string)  [unwired: 9 in]
          n160 = call "Get Variant Data Type.vi"("Variant in"=w409) -> ("first data type"=w410:string)  [unwired: 9 in, 1 out]
          n161 = Concatenate Strings(w412, w414, w412) -> (w415:string)
          n162 = Equal?(x=w410, y="String") -> (x = y?=w413:bool)
          n163 = Select(t=w415, s=w413, f=w414) -> (s? t:f=w407:string)
          n164 = To Variant(anything=w407) -> (Variant=w408:variant)
        }
        frame "Tunnel" {
          w425 = refnum<vi> refnum  # Tunnel
          # "Getting name of wire connected to Outside Terminal, because we are only interested in wires which contain INPUT values."
          n165 = To More Specific Class(target class=w425, reference=w423) -> (specific class reference=w422:refnum<vi>)  [unwired: 1 in, 1 out]
          n166 = property class="Tun"(reference=w422) -> ("Outer Term"=w421:refnum<vi>)  [unwired: 1 in, 2 out]
          n167 = property class="OutrTerm"(reference=w421) -> ("Wire"=w420:refnum<vi>)  [unwired: 1 in, 2 out]
          n168 = call "Get Wire Info.vi"("Wire"=w420) -> ("wire label"=w419:string)  [unwired: 9 in, 1 out]
          n169 = To Variant(anything=w419) -> (Variant=w424:variant)
        }
      }
      n170 = case shown="Default" w374 {
        tunnel: [w386 w387] -> w379
        tunnel: w378 -> [w386 _]
        tunnel: w377 -> [_ w389]
        frame Default {
          # "For all others Terminal.Owner don't need to do anything else."
        }
        frame "Tunnel" {
          w391 = refnum<vi> refnum  # Tunnel
          # "Creating declarations for Tunnel terminals which are IN."
          n171 = To More Specific Class(target class=w391, reference=w389) -> (specific class reference=w392:refnum<vi>)  [unwired: 1 in, 1 out]
          n172 = property class="Tun"(reference=w392) -> ("Outer Term"=w390:refnum<vi>)  [unwired: 1 in, 2 out]
          n173 = property class="OutrTerm"(reference=w390) -> ("IsSource"=w388:bool)  [unwired: 1 in, 2 out]
          n174 = Not(x=w388) -> (.not. x?=w387:bool)
        }
      }
    }
    n175 = call "Get Wire Info.vi"("Wire"=w360) -> ("wire datatype"=w356:string, "wire label"=w358:string)  [unwired: 9 in]
    n176 = Index Array(array=w361) -> (element=w352:variant)  [unwired: 1 in]
    n177 = call "Get Variant Value.vi"("Variant in"=w352) -> ("Variant value as string"=w351:string)  [unwired: 10 in]
    n178 = Empty String/Path?(string/path=w351) -> (empty?=w359:bool)
    n179 = call "LabVIEW Datatype Prefix.vi"() -> ("datatype prefix"=w348:string)
    n180 = Not(x=w359) -> (.not. x?=w354:bool)
    n181 = case shown="True" w354 {
      tunnel: w358 -> [w365 w370]
      tunnel: w356 -> [w364 w369]
      tunnel: w351 -> [_ w372]
      tunnel: [w366 w371] -> w357
      tunnel: w348 -> [w363 w368]
      frame False {
        # "If wire not connected just make declaration."
        n182 = Format Into String(format string="%s%s %s;", w363, w364, w365) -> (resulting string=w366:string)  [unwired: 2 in, 1 out]
      }
      frame True {
        # "If wire connected to Constant or some value assign it."
        n183 = Format Into String(format string="%s%s %s = %s;", w368, w369, w370, w372) -> (resulting string=w371:string)  [unwired: 2 in, 1 out]
      }
    }
    n184 = Not Equal?(x=w356, y="error") -> (x != y?=w353:bool)
  }
  "Diagram wires declarations" <- w56
  n185 = Index Array(array=w23) -> (element=w22:string)  [unwired: 1 in]
  n186 = Format Into String(format string="return %s;", w22) -> (resulting string=w19:string)  [unwired: 2 in, 1 out]
  n187 = call "String Array Concatenate To String.vi"("insert last delimiter?"=TRUE, "Delimiter char"="\r\n", "Array String In"=w25) -> ("String"=w20:string)  [unwired: 8 in]
  n188 = Concatenate Strings(w20, "\r\n", w19) -> (w16:string)
  n189 = call "String Array Concatenate To String.vi"("insert last delimiter?"=FALSE, "Delimiter char"="\r\n", "Array String In"=w56) -> ("String"=w4:string)  [unwired: 8 in]
  n190 = call "String Array Concatenate To String.vi"("insert last delimiter?"=FALSE, "Delimiter char"="\r\n", "Array String In"=w61) -> ("String"=w55:string)  [unwired: 8 in]
  n191 = call "String Array Concatenate To String.vi"("insert last delimiter?"=FALSE, "Delimiter char"="\r\n", "Array String In"=w37) -> ("String"=w3:string)  [unwired: 8 in]
  n192 = call "Unbundle Code Cluster.vi"("code chunks cluster"=w15) -> ("Defines"=w32:string[], "Includes"=w36:string[])  [unwired: 8 in, 1 out]
  n193 = property class="Diag"(reference=w13) -> ("Owner"=w12:refnum<vi>)  [unwired: 1 in, 2 out]
  n194 = property class="Gen"(reference=w12) -> (error out=w11:errorcluster, "ClassName"=w9:string)  [unwired: 1 in, 1 out]
  n195 = call "String Array Delete Duplicates.vi"("Array"=w36) -> ("Output array"=w35:string[])
  n196 = Unbundle By Name(w11) -> ("status"=w10:bool)
  n197 = Not(x=w10) -> (.not. x?=w7:bool)
  n198 = Equal?(x=w9, y="CaseStructure") -> (x = y?=w6:bool)
  n199 = And(x=w7, y=w6) -> (x .and. y?=w5:bool)
  n200 = case shown="True" w5 {
    tunnel: w3 -> [w427 w431]
    tunnel: w4 -> [w426 w430]
    tunnel: [w428 w429] -> w2
    tunnel: [w426 _] -> w1
    frame False {
      # "Default, all except CaseStructure"
      n201 = Build Array(w427) -> (w428:string[])
    }
    frame True {
      # "CaseStructure:\n- wires declaration in defines"
      n202 = Build Array(w431, w430) -> (w429:string[])
    }
  }
  n203 = Build Array(w1, w55) -> (w45:string[])
  n204 = call "String Array Concatenate To String.vi"("insert last delimiter?"=FALSE, "Delimiter char"="\r\n", "Array String In"=w45) -> ("String"=w43:string)  [unwired: 8 in]
  n205 = call "String Replace LabVIEW Data Types With C types.vi"("C code"=w43) -> ("C code, replaced datatypes"=w18:string)
  n206 = Build Array (concatenate)(w2, w32) -> (w33:string[])
  n207 = case shown="True" w10 {
    tunnel: w18 -> [w432 w436]
    tunnel: [w432 w435] -> w17
    tunnel: w16 -> [_ w434]
    frame False {
      # "Owner of Diagram is Loop or something else, don't do retur ...; assignement."
    }
    frame True {
      # "Owner of Diagram is SubVI, so doing return assignement."
      n208 = Concatenate Strings(w436, "\r\n", w434) -> (w435:string)
    }
  }
  "transcripted code" <- w17
  n209 = call "String Array Delete Duplicates.vi"("Array"=w33) -> ("Output array"=w34:string[])
  n210 = Bundle By Name(cluster=T1 {"Defines"=[], "Includes"=[], "C code"=""} ("input cluster"), "Includes"=w35, "Defines"=w34, "C code"=w17) -> (→"output cluster":T1)
